vi "H+_estimate.vi"(1 "k":dbl, 2 "EO Estimate":dbl, 3 "EMFs (pH3-3.5)":dbl[](array[numeric])) -> (0 "H+ Estimate":dbl[](array[numeric]))   [LabVIEW 2010]
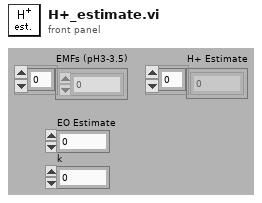
[diagram p1: front panel]
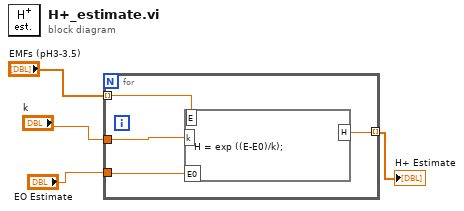
[diagram p0: block diagram]
diagram:
  n1 = for {
    tunnel: [w8] -> w4 mode=indexing
    tunnel: "EO Estimate" -> [w7]
    tunnel: "EMFs (pH3-3.5)" -> [w5] mode=indexing
    tunnel: "k" -> [w6]
    n2 = formula code="H = exp ((E-E0)/k);"("E0"=w7, "E"=w5, "k"=w6) -> ("H"=w8:dbl)
  }
  "H+ Estimate" <- w4
